vi "Delete Cell.vi"(8 "error in (no error)":errorcluster, 11 "Run Block in":refnum<class "Run Block.lvclass">) -> (0 "error out":errorcluster, 3 "Run Block out":refnum<class "Run Block.lvclass">)   [LabVIEW 2020, in "Run Utilities.lvlib" / "Run Block.lvclass"]
doc: "Delete a cell from the schedule based on the inner index selector. The selector can be specified via the <b>Select Cell.vi</b> (or Index selector property node)."
uses:
  Run Block.lvclass
  Run Block.lvclass/Run Block.ctl
  Schedule/Schedule.lvclass
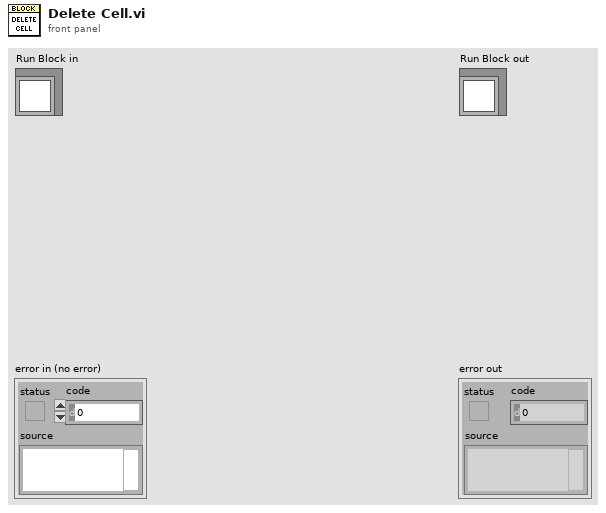
[diagram p1: front panel]
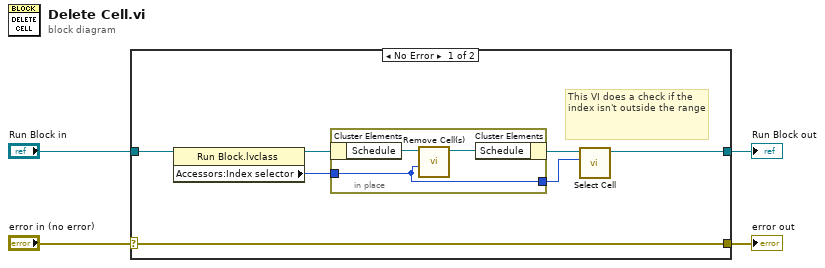
[diagram p0: block diagram]
diagram:
  n1 = case shown="No Error" "error in (no error)" {
    selector: "error in (no error)" -> [w11 w16]
    tunnel: [w11 w16] -> w3
    tunnel: [w6 w15] -> w1
    tunnel: "Run Block in" -> [w10 w15]
    frame No Error {
      # "This VI does a check if the index isn't outside the range"
      n2 = property class="Run Block.lvclass"(reference=w10) -> (reference out=w9:refnum<class "Run Block.lvclass">, "Accessors:Index selector"=w8:i32)  [unwired: 1 in, 1 out]
      n3 = in-place {
        in-place-border: w8 -> [w12]
        in-place-border: [w12] -> w5
        n4 = in-place-cluster #1(w9) -> ("Schedule"=w14:refnum<class "Schedule.lvclass">)
        n5 = call-dynamic "Remove Cell(s).vi"("index"=w12, "Schedule in"=w14) -> ("Schedule out"=w13:refnum<class "Schedule.lvclass">)  [unwired: 7 in, 2 out]
        n6 = in-place-cluster #1("Schedule"=w13) -> (w7:refnum<class "Run Block.lvclass">)
      }
      n7 = call-dynamic "Select Cell.vi"("Index selector"=w5, "Run Block in"=w7) -> ("Run Block out"=w6:refnum<class "Run Block.lvclass">)  [unwired: 8 in, 1 out]
    }
    frame Error {
    }
  }
  "error out" <- w3
  "Run Block out" <- w1
